vi "FindParentActorAttributes.vi"(11 "Actor":refnum<class "Actor.lvclass">) -> (3 "ParentActorAttributes":T1)   [LabVIEW 2020, in "jettl.lvlib"]
uses:
  jettl.lvlib
  Actor/Actor.lvclass
  Msg/Msg.lvclass
  MsgNames.ctl
  Msg.ctl
  PostSetup.ctl
  PreSetup.ctl
  ActorAttribs.ctl
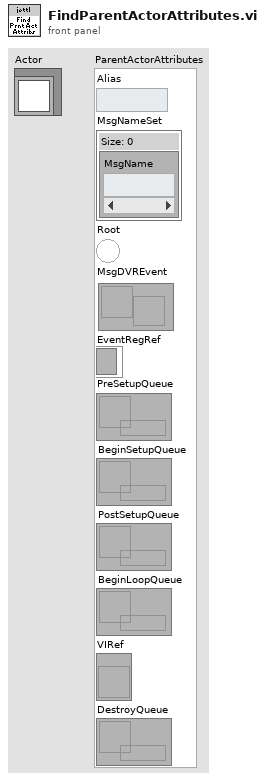
[diagram p1: front panel]
types:
  T1 = typedef "jettl.lvlib/ActorAttribs.ctl" = cluster{"Alias":string, "MsgNameSet":T2, "Root":bool, "MsgDVREvent":refnum<user-event>, "EventRegRef":refnum<event-registration>, "PreSetupQueue":refnum<queue>, "BeginSetupQueue":refnum<queue>, "PostSetupQueue":refnum<queue>, "BeginLoopQueue":refnum<queue>, "VIRef":refnum<vi>, "DestroyQueue":refnum<queue>}
  T2 = typedef "jettl.lvlib/MsgNames.ctl" = set{string}
  T3 = typedef "jettl.lvlib/UnifiedAttribs.ctl" = cluster{"State":T4, "SelfActor":T1, "ParentActor":T1, "ChildActors":T6}
  T4 = typedef "jettl.lvlib/State.ctl" = cluster{"Lifecycle":T5, "BeganLoop":bool}
  T5 = typedef "jettl.lvlib/Lifecycle.ctl" = enum16{"Initializing", "SettingUp", "Starting", "Running", "Stopping", "TearingDown", "Terminated"}
  T6 = typedef "jettl.lvlib/ChildActors.ctl" = map{string, T1}
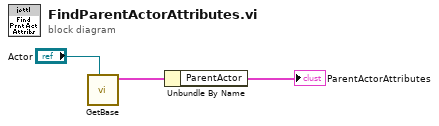
[diagram p0: block diagram]
diagram:
  n1 = call-dynamic "GetBase.vi"("Actor"="Actor") -> ("Base"=w2:T3)  [unwired: 10 in]
  n2 = Unbundle By Name(w2) -> ("ParentActor"=→"ParentActorAttributes":T1)
